vi "test-path-planner-sample.vi"() -> ()   [LabVIEW 2019]
uses:
  <vilib>/Rock Robotics/WPI/ThirdParty/MJansen/PathPlanner/PathPlanner24.lvlib
  <vilib>/Rock Robotics/WPI/ThirdParty/JAS_Junk/TrajLib/Trajectory_Library.lvlib
  <vilib>/Analysis/NI_AALBase.lvlib
  <vilib>/Rock Robotics/WPI/ThirdParty/JAS_Junk/TrajLib/TypeDef/ROTATION2D.ctl
  <vilib>/Rock Robotics/WPI/ThirdParty/JAS_Junk/TrajLib/TypeDef/TRANSLATION2D.ctl
  <vilib>/Rock Robotics/WPI/ThirdParty/MJansen/PathPlanner/TypeDef/PathPlannerTrajectoryState.ctl
  <vilib>/Rock Robotics/WPI/ThirdParty/MJansen/PathPlanner/TypeDef/PathPlannerTrajectory.ctl
  <vilib>/Rock Robotics/WPI/ThirdParty/MJansen/PathPlanner/TypeDef/PathPlannerPathConstraints.ctl
  <vilib>/Rock Robotics/WPI/ThirdParty/JAS_Junk/TrajLib/TypeDef/POSE2D.ctl
  <vilib>/Rock Robotics/WPI/ThirdParty/JAS_Junk/TrajLib/TypeDef/TRAJ_STATE.ctl
  <vilib>/Rock Robotics/WPI/ThirdParty/MJansen/PathPlanner/TypeDef/PathPlannerWaypoint.ctl
panel:
  in  "Tab Control":T1(tab)
  in  "Max Velocity":dbl=3.0
  in  "Max Acceleration":dbl=2.0
  in  "stop":bool
  in  "Reversed":bool
  out "PathPlannerWayPoints":T2[](array[typedef]) {"nextControl"."Y" format="%14.3f"; "nextControl"."X" format="%14.3f"; "anchor"."Y" format="%14.3f"; "anchor"."X" format="%14.3f"; "prevControl"."Y" format="%14.3f"; "prevControl"."X" format="%14.3f"}
  in  "Path FileName":string="C:\\Shares\\github\\PathPlannerLabVIEW\\PathPlannerSandbox\\PathPlannerTestPath\\JIM1.path"
  out "LabVIEW path json read error":errorcluster
  out "PathPlannerTrajectory":T4 {"States"."TargetHolonomicRotation"."SIN" format="%13.4f"; "States"."TargetHolonomicRotation"."COS" format="%13.4f"; "States"."TargetHolonomicRotation"."VALUE" format="%13.4f"; "States"."Heading"."SIN" format="%13.4f"; "States"."Heading"."COS" format="%13.4f"; "States"."Heading"."VALUE" format="%13.4f"; "States"."PositionMeters"."Y" format="%14.3f"; "States"."PositionMeters"."X" format="%14.3f"}
  out "outPathPlannerStates":T5[](array[typedef]) {"TargetHolonomicRotation"."SIN" format="%13.4f"; "TargetHolonomicRotation"."COS" format="%13.4f"; "TargetHolonomicRotation"."VALUE" format="%13.4f"; "Heading"."SIN" format="%13.4f"; "Heading"."COS" format="%13.4f"; "Heading"."VALUE" format="%13.4f"; "PositionMeters"."Y" format="%14.3f"; "PositionMeters"."X" format="%14.3f"}
  in  "index":i32
  out "LabVIEW_TotalTime_Sec":dbl
  out "LabVIEWStateCount":i32
  out "States Check":bool[](array[boolean])
  out "Differences":T8[](array[typedef]) {"POSE"."ROTATION"."SIN" format="%13.4f"; "POSE"."ROTATION"."COS" format="%13.4f"; "POSE"."ROTATION"."VALUE" format="%13.4f"; "POSE"."TRANSLATION"."Y" format="%14.3f"; "POSE"."TRANSLATION"."X" format="%14.3f"}
  out "max time diff":dbl
  out "max vel diff":dbl
  out "max accel diff":dbl
  out "max x diff":dbl
  out "max y diff":dbl
  out "max rot diff rad":dbl
  out "max curvature diff":dbl
  out "vel mean":dbl format="%0.6f"
  out "vel std dev":dbl format="%0.6f"
  out "accel mean":dbl format="%0.6f"
  out "accel std dev":dbl format="%0.6f"
  out "Java and LabVIEW \nwithin tolerance":bool
  out "max accel diff\nindex":i32
  out "max time diff\nindex":i32
  out "Path Samp":T8[](array[typedef]) {"POSE"."ROTATION"."SIN" format="%13.4f"; "POSE"."ROTATION"."COS" format="%13.4f"; "POSE"."ROTATION"."VALUE" format="%13.4f"; "POSE"."TRANSLATION"."Y" format="%14.3f"; "POSE"."TRANSLATION"."X" format="%14.3f"}
  out "LV Samp":T8[](array[typedef]) {"POSE"."ROTATION"."SIN" format="%13.4f"; "POSE"."ROTATION"."COS" format="%13.4f"; "POSE"."ROTATION"."VALUE" format="%13.4f"; "POSE"."TRANSLATION"."Y" format="%14.3f"; "POSE"."TRANSLATION"."X" format="%14.3f"}
  in  "Tolerance":T8={"TimeSeconds"=0.005, "Velocity"=0.005, "Acceleration"=0.2, "POSE"={"TRANSLATION"={"X"=0.002, "Y"=0.002}, "ROTATION"={"VALUE"=0.002, "COS"=0.002, "SIN"=0.002}}, "Curvature"=0.3} {"POSE"."ROTATION"."SIN" format="%13.4f"; "POSE"."ROTATION"."COS" format="%13.4f"; "POSE"."ROTATION"."VALUE" format="%13.4f"; "POSE"."TRANSLATION"."Y" format="%14.3f"; "POSE"."TRANSLATION"."X" format="%14.3f"}
  out "XY SPLINE":cluster{dbl[], dbl[]}[](graph)
  out "XY Graph":cluster{dbl[], dbl[]}[](graph)
  out "Sample Graph":dbl[][](graph)
  out "LabVIEW Time Plot":cluster{dbl[], dbl[]}[](graph)
  out "Diff Time Plot":cluster{dbl[], dbl[]}[](graph)
  in  "PPS2":T5={"TimeSeconds"=4.0, "VelocityMPS"=4.0, "AccerationMpsSq"=4.0, "HeadingAngularVelRadPerSec"=4.0, "PositionMeters"={"X"=1.5, "Y"=0.071}, "Heading"={"VALUE"=1.5, "COS"=0.071, "SIN"=0.997}, "TargetHolonomicRotation"={"VALUE"=0.0, "COS"=1.0, "SIN"=0.0}, "CurvatureRadPerMeter"=4.0, "PathPlannerConstraints"={"MaxVelocityMps;"=2.0, "MaxAccelerationMpsSq;"=4.0, "MaxAngularVelRadPsEc;"=4.0, "MaxAngularAccRadPSecSq"=0.25, "Exists"=FALSE, "Unlimited"=FALSE, "NominalVoltageVolts"=1.5}, "DeltaPos"=2.0} {"TargetHolonomicRotation"."SIN" format="%13.4f"; "TargetHolonomicRotation"."COS" format="%13.4f"; "TargetHolonomicRotation"."VALUE" format="%13.4f"; "Heading"."SIN" format="%13.4f"; "Heading"."COS" format="%13.4f"; "Heading"."VALUE" format="%13.4f"; "PositionMeters"."Y" format="%14.3f"; "PositionMeters"."X" format="%14.3f"}
  in  "PPS1":T5={"TimeSeconds"=2.0, "VelocityMPS"=2.0, "AccerationMpsSq"=2.0, "HeadingAngularVelRadPerSec"=2.0, "PositionMeters"={"X"=0.5, "Y"=0.878}, "Heading"={"VALUE"=0.5, "COS"=0.878, "SIN"=0.479}, "TargetHolonomicRotation"={"VALUE"=0.0, "COS"=1.0, "SIN"=0.0}, "CurvatureRadPerMeter"=2.0, "PathPlannerConstraints"={"MaxVelocityMps;"=1.0, "MaxAccelerationMpsSq;"=2.0, "MaxAngularVelRadPsEc;"=2.0, "MaxAngularAccRadPSecSq"=0.5, "Exists"=FALSE, "Unlimited"=FALSE, "NominalVoltageVolts"=0.5}, "DeltaPos"=1.0} {"TargetHolonomicRotation"."SIN" format="%13.4f"; "TargetHolonomicRotation"."COS" format="%13.4f"; "TargetHolonomicRotation"."VALUE" format="%13.4f"; "Heading"."SIN" format="%13.4f"; "Heading"."COS" format="%13.4f"; "Heading"."VALUE" format="%13.4f"; "PositionMeters"."Y" format="%14.3f"; "PositionMeters"."X" format="%14.3f"}
  in  "PPS0":T5={"TimeSeconds"=1.0, "VelocityMPS"=1.0, "AccerationMpsSq"=1.0, "HeadingAngularVelRadPerSec"=1.0, "PositionMeters"={"X"=0.0, "Y"=1.0}, "Heading"={"VALUE"=0.0, "COS"=1.0, "SIN"=0.0}, "TargetHolonomicRotation"={"VALUE"=0.0, "COS"=1.0, "SIN"=0.0}, "CurvatureRadPerMeter"=1.0, "PathPlannerConstraints"={"MaxVelocityMps;"=0.0, "MaxAccelerationMpsSq;"=1.0, "MaxAngularVelRadPsEc;"=1.0, "MaxAngularAccRadPSecSq"=1.0, "Exists"=FALSE, "Unlimited"=FALSE, "NominalVoltageVolts"=0.0}, "DeltaPos"=1.0} {"TargetHolonomicRotation"."SIN" format="%13.4f"; "TargetHolonomicRotation"."COS" format="%13.4f"; "TargetHolonomicRotation"."VALUE" format="%13.4f"; "Heading"."SIN" format="%13.4f"; "Heading"."COS" format="%13.4f"; "Heading"."VALUE" format="%13.4f"; "PositionMeters"."Y" format="%14.3f"; "PositionMeters"."X" format="%14.3f"}
  out "TrajState":T8={"TimeSeconds"=0.0, "Velocity"=0.0, "Acceleration"=0.0, "POSE"={"TRANSLATION"={"X"=0.0, "Y"=0.0}, "ROTATION"={"VALUE"=0.0, "COS"=1.0, "SIN"=0.0}}, "Curvature"=0.0} {"POSE"."ROTATION"."SIN" format="%13.4f"; "POSE"."ROTATION"."COS" format="%13.4f"; "POSE"."ROTATION"."VALUE" format="%13.4f"; "POSE"."TRANSLATION"."Y" format="%14.3f"; "POSE"."TRANSLATION"."X" format="%14.3f"}
  out "PathState":T8={"TimeSeconds"=0.0, "Velocity"=0.0, "Acceleration"=0.0, "POSE"={"TRANSLATION"={"X"=0.0, "Y"=0.0}, "ROTATION"={"VALUE"=0.0, "COS"=1.0, "SIN"=0.0}}, "Curvature"=0.0} {"POSE"."ROTATION"."SIN" format="%13.4f"; "POSE"."ROTATION"."COS" format="%13.4f"; "POSE"."ROTATION"."VALUE" format="%13.4f"; "POSE"."TRANSLATION"."Y" format="%14.3f"; "POSE"."TRANSLATION"."X" format="%14.3f"}
  out "LabVIEWStates":T8[](array[typedef]) {"POSE"."ROTATION"."SIN" format="%13.4f"; "POSE"."ROTATION"."COS" format="%13.4f"; "POSE"."ROTATION"."VALUE" format="%13.4f"; "POSE"."TRANSLATION"."Y" format="%14.3f"; "POSE"."TRANSLATION"."X" format="%14.3f"}
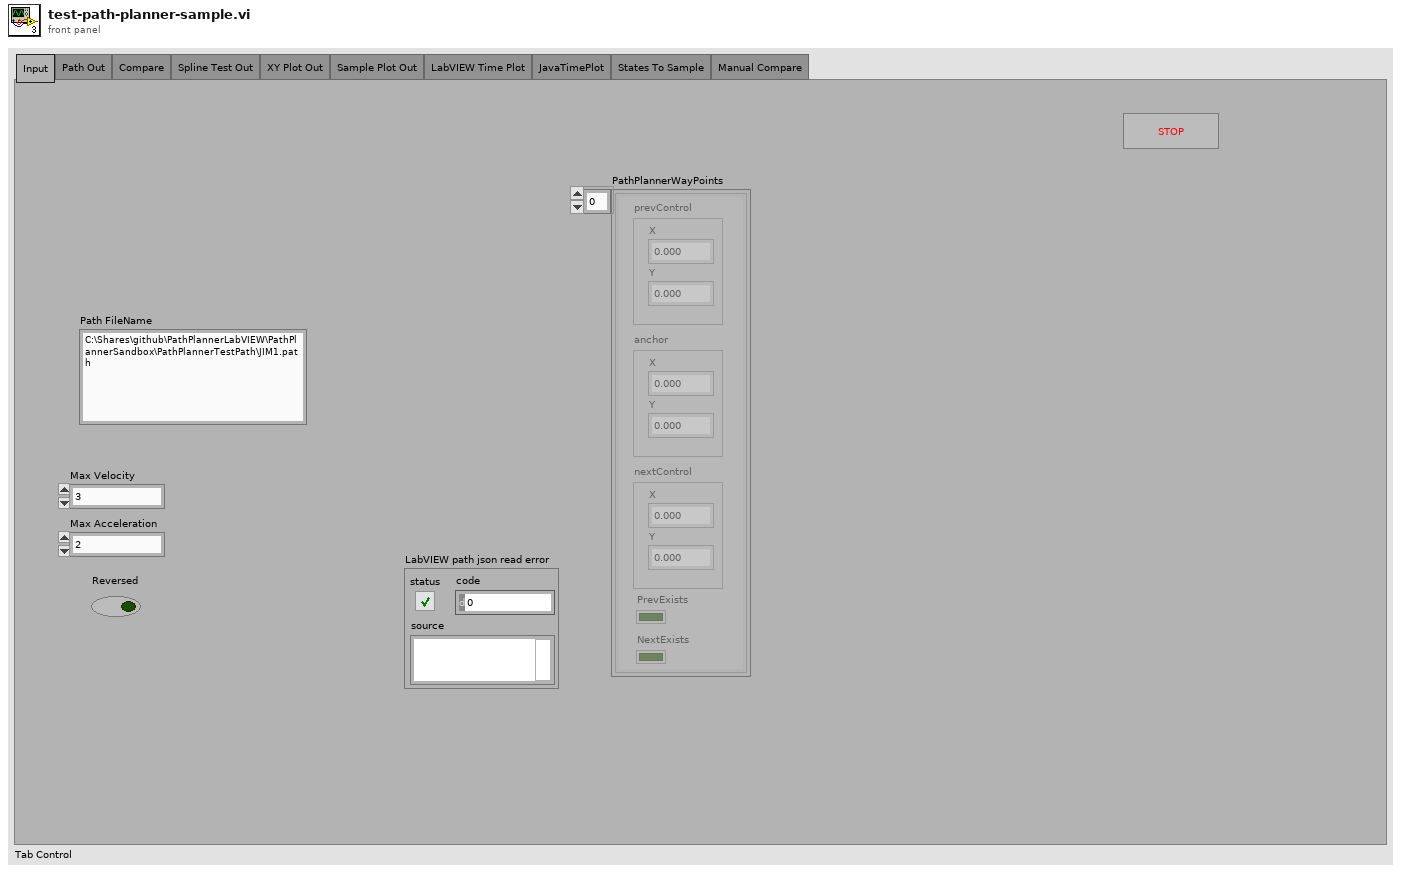
[diagram p1: front panel]
types:
  T1 = enum32{"Input", "Path Out", "Compare", "Spline Test Out", "XY Plot Out", "Sample Plot Out", "LabVIEW Time Plot", "JavaTimePlot", "States To Sample", "Manual Compare"}
  T2 = typedef "PathPlanner24.lvlib/PathPlannerWaypoint.ctl" = cluster{"prevControl":T3, "anchor":T3, "nextControl":T3, "PrevExists":bool, "NextExists":bool}
  T3 = typedef "Trajectory_Library.lvlib/TRANSLATION2D.ctl" = cluster{"X":dbl, "Y":dbl}
  T4 = typedef "PathPlanner24.lvlib/PathPlannerTrajectory.ctl" = cluster{"States":T5[]}
  T5 = typedef "PathPlanner24.lvlib/PathPlannerTrajectoryState.ctl" = cluster{"TimeSeconds":dbl, "VelocityMPS":dbl, "AccerationMpsSq":dbl, "HeadingAngularVelRadPerSec":dbl, "PositionMeters":T3, "Heading":T6, "TargetHolonomicRotation":T6, "CurvatureRadPerMeter":dbl, "PathPlannerConstraints":T7, "DeltaPos":dbl}
  T6 = typedef "Trajectory_Library.lvlib/ROTATION2D.ctl" = cluster{"VALUE":dbl, "COS":dbl, "SIN":dbl}
  T7 = typedef "PathPlanner24.lvlib/PathPlannerPathConstraints.ctl" = cluster{"MaxVelocityMps;":dbl, "MaxAccelerationMpsSq;":dbl, "MaxAngularVelRadPsEc;":dbl, "MaxAngularAccRadPSecSq":dbl, "Exists":bool, "Unlimited":bool, "NominalVoltageVolts":dbl}
  T8 = typedef "Trajectory_Library.lvlib/TRAJ_STATE.ctl" = cluster{"TimeSeconds":dbl, "Velocity":dbl, "Acceleration":dbl, "POSE":T9, "Curvature":dbl}
  T9 = typedef "Trajectory_Library.lvlib/POSE2D.ctl" = cluster{"TRANSLATION":T3, "ROTATION":T6}
  T10 = typedef "Trajectory_Library.lvlib/TRAJECTORY.ctl" = cluster{"TotalTImeSecs":dbl, "States":T8[]}
  T11 = typedef "PathPlanner24.lvlib/PathPlannerPath.ctl" = cluster{"Reversed":bool, "RotationTargets":T12[], "ConstraintZones":T13[], "EventMarkers":T14[], "GlobalConstraints":T7, "GoalEndState":T17, "AllPoints":T18[], "Name":string, "Waypoints":T2[], "PointTowardsZones":T19[], "IdealStartingState":T20, "IsChoreoPath":bool, "PreventFlipping":bool}
  T12 = typedef "PathPlanner24.lvlib/PathPlannerRotationTarget.ctl" = cluster{"position":dbl, "rotation":T6, "Exists":bool}
  T13 = typedef "PathPlanner24.lvlib/PathPlannerConstraintsZone.ctl" = cluster{"minPosition":dbl, "maxPosition":dbl, "Constraints":T7, "Present":bool}
  T14 = typedef "PathPlanner24.lvlib/PathPlannerEventMarker.ctl" = cluster{"Position":dbl, "Command":T15, "TriggerName":string, "EndPosition":dbl}
  T15 = typedef "PathPlanner24.lvlib/PathPlannerCommandUtil.ctl" = cluster{"waitTime":dbl, "name":string, "pathName":string, "commands":cluster{"type":T16, "waitTime":dbl, "name":string, "pathName":string}[], "type":T16}
  T16 = typedef "PathPlanner24.lvlib/PathPlanner_CommandUtilType_ENUM.ctl" = enum16{"Unknown", "Wait", "Named", "Path", "Sequential", "Parallel", "Race", "Deadline"}
  T17 = typedef "PathPlanner24.lvlib/PathPlannerGoalEndState.ctl" = cluster{"VelocityMPS":dbl, "Rotation":T6}
  T18 = typedef "PathPlanner24.lvlib/PathPlannerPathPoint.ctl" = cluster{"Position":T3, "DistAlongPath":dbl, "MaxV":dbl, "Constraints":T7, "RotationTarget":T12, "WaypointRelativePos":dbl}
  T19 = typedef "PathPlanner24.lvlib/PathPlannerPointTowardsZone.ctl" = cluster{"RotationOffset":T6, "Name":string, "TargetPosition":T3, "MinPosition":dbl, "MaxPosition":dbl}
  T20 = typedef "PathPlanner24.lvlib/PathPlannerIdealStartingState.ctl" = cluster{"VelocityMPS":dbl, "Rotation":T6}
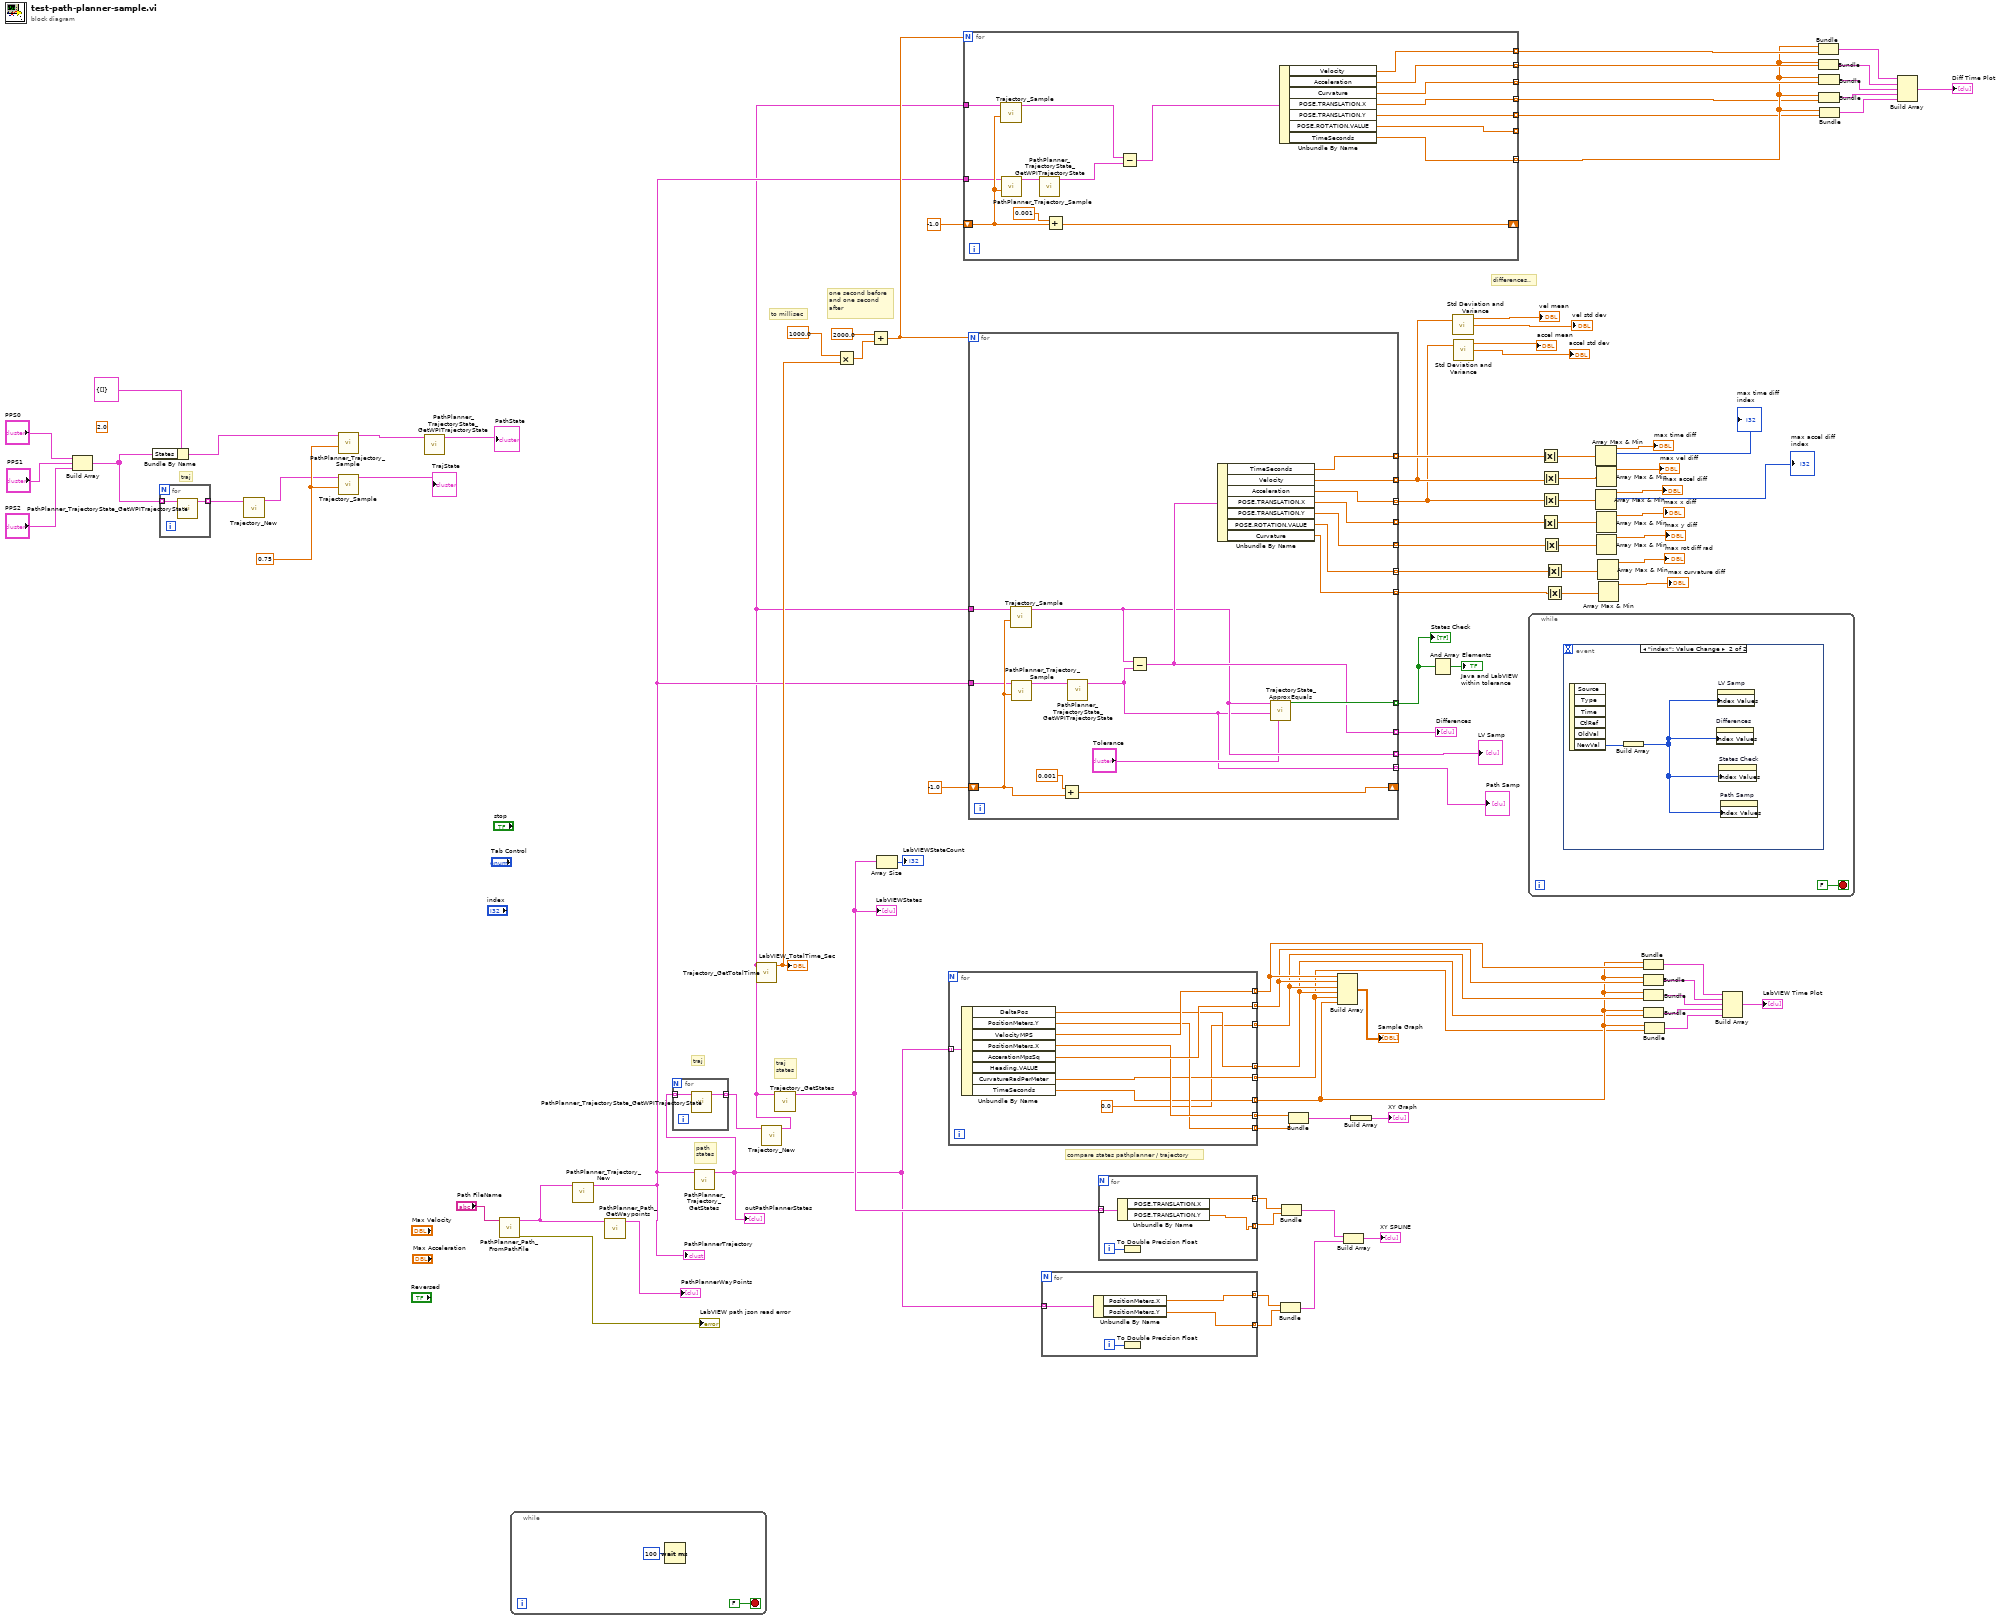
[diagram p0: block diagram]
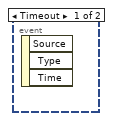
[diagram p2: hidden frame]
diagram:
  w18 = 0.75
  (unwired) 2.0 ("TotalTimeSeconds")
  # "traj"
  # "one second before\nand one second\nafter"
  # "to millisec"
  # "compare states pathplanner / trajectory"
  # "traj"
  # "traj\nstates"
  # "path\nstates"
  # "differences.."
  n1 = Build Array("PPS0", "PPS1", "PPS2") -> (w5:T5[])
  n2 = Bundle By Name(cluster=T4 {"States"=[]} ("PathPlannerTrajectory"), "States"=w5) -> (w6:T4)
  n3 = for {
    tunnel: w5 -> [w99] mode=indexing
    tunnel: [w98] -> w4 mode=indexing
    n4 = call <vilib>:"PathPlanner_TrajectoryState_GetWPITrajectoryState.vi"("PathPlannerState"=w99) -> ("WPI TrajectoryState"=w98:T8)  [unwired: 9 in, 1 out]
  }
  n5 = call <vilib>:"Trajectory_New.vi"("TRAJ_STATES"=w4) -> ("TRAJECTORY"=w3:T10)  [unwired: 10 in]
  n6 = call <vilib>:"PathPlanner_Trajectory_Sample.vi"("Time"=w18, "PathPlannerTrajectory"=w6) -> ("PathPlannerState"=w2:T5)  [unwired: 9 in]
  n7 = call <vilib>:"Trajectory_Sample.vi"("Time"=w18, "InputTRAJECTORY"=w3) -> ("OutputTRAJ_STATE"=→"TrajState":T8)  [unwired: 9 in]
  n8 = call <vilib>:"PathPlanner_TrajectoryState_GetWPITrajectoryState.vi"("PathPlannerState"=w2) -> ("WPI TrajectoryState"=→"PathState":T8)  [unwired: 9 in, 1 out]
  n9 = call <vilib>:"PathPlanner_Path_FromPathFile.vi"("FileName"="Path FileName") -> ("error out"=→"LabVIEW path json read error":errorcluster, "PathPlannerPath"=w11:T11)  [unwired: 7 in, 2 out]
  n10 = while {
    stop <- FALSE stop-if-true
    n11 = Wait (ms)(milliseconds to wait=u32 100) -> ()  [unwired: 1 out]
  }
  n12 = call <vilib>:"PathPlanner_Trajectory_New.vi"("Path"=w11) -> ("PathPlannerTrajectory"=w12:T4)  [unwired: 9 in, 1 out]
  "PathPlannerTrajectory" <- w12
  n13 = call <vilib>:"PathPlanner_Path_GetWaypoints.vi"("PathPlannerPath"=w11) -> ("Waypoints"=→"PathPlannerWayPoints":T2[])  [unwired: 10 in]
  n14 = call <vilib>:"PathPlanner_Trajectory_GetStates.vi"("PathPlannerTrajectory"=w12) -> ("PathPlannerStates"=w9:T5[])  [unwired: 10 in]
  "outPathPlannerStates" <- w9
  n15 = for {
    tunnel: w9 -> [w103] mode=indexing
    tunnel: [w102] -> w8 mode=indexing
    n16 = call <vilib>:"PathPlanner_TrajectoryState_GetWPITrajectoryState.vi"("PathPlannerState"=w103) -> ("WPI TrajectoryState"=w102:T8)  [unwired: 9 in, 1 out]
  }
  n17 = call <vilib>:"Trajectory_New.vi"("TRAJ_STATES"=w8) -> ("TRAJECTORY"=w7:T10)  [unwired: 10 in]
  n18 = call <vilib>:"Trajectory_GetTotalTime.vi"("TRAJECTORY"=w7) -> ("TotalTime_Sec"=w40:dbl)  [unwired: 10 in]
  "LabVIEW_TotalTime_Sec" <- w40
  n19 = call <vilib>:"Trajectory_GetStates.vi"("TRAJECTORY"=w7) -> ("States"=w41:T8[])  [unwired: 10 in]
  "LabVIEWStates" <- w41
  n20 = Multiply(x=1000.0, y=w40) -> (x*y=w44:dbl)
  n21 = Add(x=2000.0, y=w44) -> (x+y=w39:dbl)
  n22 = Array Size(array=w41) -> (size(s)=→"LabVIEWStateCount":i32)
  n23 = for {
    tunnel: [w112] -> w70 mode=indexing
    tunnel: [w111] -> w69 mode=indexing
    tunnel: [w106] -> w66 mode=indexing
    tunnel: [w110] -> w96 mode=indexing
    tunnel: [w109] -> w95 mode=indexing
    tunnel: w9 -> [w108] mode=indexing
    tunnel: [w107] -> w65 mode=indexing
    tunnel: [0.0] -> w68 mode=indexing
    tunnel: [w105] -> w67 mode=indexing
    n24 = Unbundle By Name(w108) -> ("DeltaPos"=w106:dbl, "PositionMeters.Y"=w109:dbl, "VelocityMPS"=w112:dbl, "PositionMeters.X"=w110:dbl, "AccerationMpsSq"=w111:dbl, "CurvatureRadPerMeter"=w107:dbl, "TimeSeconds"=w105:dbl)  [unwired: 1 out]
  }
  n25 = for {
    N: w39 -> [_]
    tunnel: [w120] -> w59 mode=indexing
    tunnel: [w119] -> w58 mode=indexing
    tunnel: [w117] -> w55 mode=indexing
    tunnel: [w116] -> w54 mode=indexing
    tunnel: [w118] -> w57 mode=indexing
    tunnel: [w128] -> w56 mode=indexing
    shift-right: [w124] -> _
    shift-left: -1.0 -> [w123]
    tunnel: w12 -> [w122]
    tunnel: w7 -> [w121]
    tunnel: [w115] -> _ mode=indexing
    n26 = call <vilib>:"Trajectory_Sample.vi"("Time"=w123, "InputTRAJECTORY"=w121) -> ("OutputTRAJ_STATE"=w127:T8)  [unwired: 9 in]
    n27 = call <vilib>:"PathPlanner_Trajectory_Sample.vi"("Time"=w123, "PathPlannerTrajectory"=w122) -> ("PathPlannerState"=w114:T5)  [unwired: 9 in]
    n28 = call <vilib>:"PathPlanner_TrajectoryState_GetWPITrajectoryState.vi"("PathPlannerState"=w114) -> ("WPI TrajectoryState"=w113:T8)  [unwired: 9 in, 1 out]
    n29 = Add(x=0.001, y=w123) -> (x+y=w124:dbl)
    n30 = Subtract(x=w127, y=w113) -> (x-y=w126:T8)
    n31 = Unbundle By Name(w126) -> ("Velocity"=w120:dbl, "Acceleration"=w119:dbl, "Curvature"=w118:dbl, "POSE.TRANSLATION.X"=w117:dbl, "POSE.TRANSLATION.Y"=w116:dbl, "POSE.ROTATION.VALUE"=w115:dbl, "TimeSeconds"=w128:dbl)
  }
  n32 = for {
    N: w39 -> [_]
    tunnel: [w146] -> w48 mode=indexing
    tunnel: [w145] -> w37 mode=indexing
    tunnel: [w144] -> w24 mode=indexing
    tunnel: [w143] -> w23 mode=indexing
    tunnel: [w142] -> w36 mode=indexing
    tunnel: [w141] -> w35 mode=indexing
    tunnel: [w140] -> w34 mode=indexing
    tunnel: [w139] -> w33 mode=indexing
    shift-right: [w137] -> _
    shift-left: -1.0 -> [w136]
    tunnel: w12 -> [w135]
    tunnel: w7 -> [w134]
    tunnel: [w133] -> w25 mode=indexing
    tunnel: [w132] -> w14 mode=indexing
    tunnel: [w129] -> w13 mode=indexing
    n33 = call <vilib>:"Trajectory_Sample.vi"("Time"=w136, "InputTRAJECTORY"=w134) -> ("OutputTRAJ_STATE"=w132:T8)  [unwired: 9 in]
    n34 = call <vilib>:"PathPlanner_Trajectory_Sample.vi"("Time"=w136, "PathPlannerTrajectory"=w135) -> ("PathPlannerState"=w130:T5)  [unwired: 9 in]
    n35 = Add(x=0.001, y=w136) -> (x+y=w137:dbl)
    n36 = call <vilib>:"PathPlanner_TrajectoryState_GetWPITrajectoryState.vi"("PathPlannerState"=w130) -> ("WPI TrajectoryState"=w129:T8)  [unwired: 9 in, 1 out]
    n37 = Subtract(x=w132, y=w129) -> (x-y=w133:T8)
    n38 = Unbundle By Name(w133) -> ("TimeSeconds"=w145:dbl, "Velocity"=w144:dbl, "Acceleration"=w143:dbl, "POSE.TRANSLATION.X"=w142:dbl, "POSE.TRANSLATION.Y"=w141:dbl, "POSE.ROTATION.VALUE"=w140:dbl, "Curvature"=w139:dbl)
    n39 = call "TrajectoryState_ApproxEquals.vi"("Tolerance"="Tolerance", "Other TRAJ_STATE"=w129, "TRAJ_STATE"=w132) -> ("Equals"=w146:bool)  [unwired: 8 in]
  }
  "States Check" <- w48
  "Differences" <- w25
  "LV Samp" <- w14
  "Path Samp" <- w13
  n40 = for {
    tunnel: [w149] -> w90 mode=indexing
    tunnel: w9 -> [w148] mode=indexing
    tunnel: [w147] -> w89 mode=indexing
    i -> [w150]
    n41 = Unbundle By Name(w148) -> ("PositionMeters.X"=w149:dbl, "PositionMeters.Y"=w147:dbl)
    n42 = To Double Precision Float(number=w150) -> ()  [unwired: 1 out]
  }
  n43 = for {
    tunnel: [w153] -> w92 mode=indexing
    tunnel: [w152] -> w91 mode=indexing
    tunnel: w41 -> [w151] mode=indexing
    i -> [w154]
    n44 = Unbundle By Name(w151) -> ("POSE.TRANSLATION.X"=w153:dbl, "POSE.TRANSLATION.Y"=w152:dbl)
    n45 = To Double Precision Float(number=w154) -> ()  [unwired: 1 out]
  }
  n46 = Bundle(w90, w89) -> (w87:cluster{dbl[], dbl[]})  [unwired: 1 in]
  n47 = Bundle(w92, w91) -> (w88:cluster{dbl[], dbl[]})  [unwired: 1 in]
  n48 = Bundle(w96, w95) -> (w94:cluster{dbl[], dbl[]})  [unwired: 1 in]
  n49 = Build Array(w70, w69, w68, w66, w65, w67) -> (→"Sample Graph":dbl[][])
  n50 = Build Array(w88, w87) -> (→"XY SPLINE":cluster{dbl[], dbl[]}[])
  n51 = Build Array(w94) -> (→"XY Graph":cluster{dbl[], dbl[]}[])
  n52 = And Array Elements(Boolean array=w48) -> (logical AND=→"Java and LabVIEW \nwithin tolerance":bool)
  n53 = call <vilib>:"Std Deviation and Variance.vi"("X"=w24) -> ("mean"=→"vel mean":dbl, "standard deviation"=→"vel std dev":dbl)  [unwired: 1 in, 1 out]
  n54 = call <vilib>:"Std Deviation and Variance.vi"("X"=w23) -> ("mean"=→"accel mean":dbl, "standard deviation"=→"accel std dev":dbl)  [unwired: 1 in, 1 out]
  n55 = while {
    stop <- FALSE stop-if-true
    n56 = event shown="[1] \"index\": Value Change" {
      selector: _ -> [_ _]
      dyn-events: _ -> [_ _]
      timeout: _ -> [_ _]
      event Timeout {
        n57 = event-data() -> ()  [unwired: 1 in, 3 out]
      }
      event "index": Value Change {
        n58 = event-data() -> ("NewVal"=w157:i32)  [unwired: 1 in, 5 out]
        n59 = Build Array(w157) -> (w156:i32[])
        n60 = property on="Differences" class="Arr (strict)"("Index Values"=w156) -> ()  [unwired: 2 in, 2 out]
        n61 = property on="LV Samp" class="Arr (strict)"("Index Values"=w156) -> ()  [unwired: 2 in, 2 out]
        n62 = property on="States Check" class="Arr (strict)"("Index Values"=w156) -> ()  [unwired: 2 in, 2 out]
        n63 = property on="Path Samp" class="Arr (strict)"("Index Values"=w156) -> ()  [unwired: 2 in, 2 out]
      }
    }
  }
  n64 = Absolute Value(x=w37) -> (abs(x)=w32:dbl[])
  n65 = Absolute Value(x=w36) -> (abs(x)=w29:dbl[])
  n66 = Absolute Value(x=w24) -> (abs(x)=w31:dbl[])
  n67 = Absolute Value(x=w23) -> (abs(x)=w30:dbl[])
  n68 = Absolute Value(x=w35) -> (abs(x)=w28:dbl[])
  n69 = Absolute Value(x=w34) -> (abs(x)=w27:dbl[])
  n70 = Absolute Value(x=w33) -> (abs(x)=w26:dbl[])
  n71 = Array Max & Min(array=w32) -> (max value=→"max time diff":dbl, max index (indices)=→"max time diff\nindex":i32)  [unwired: 2 out]
  n72 = Array Max & Min(array=w30) -> (max value=→"max accel diff":dbl, max index (indices)=→"max accel diff\nindex":i32)  [unwired: 2 out]
  n73 = Array Max & Min(array=w31) -> (max value=→"max vel diff":dbl)  [unwired: 3 out]
  n74 = Array Max & Min(array=w29) -> (max value=→"max x diff":dbl)  [unwired: 3 out]
  n75 = Array Max & Min(array=w28) -> (max value=→"max y diff":dbl)  [unwired: 3 out]
  n76 = Array Max & Min(array=w27) -> (max value=→"max rot diff rad":dbl)  [unwired: 3 out]
  n77 = Array Max & Min(array=w26) -> (max value=→"max curvature diff":dbl)  [unwired: 3 out]
  n78 = Bundle(w67, w70) -> (w64:cluster{dbl[], dbl[]})  [unwired: 1 in]
  n79 = Bundle(w67, w69) -> (w63:cluster{dbl[], dbl[]})  [unwired: 1 in]
  n80 = Bundle(w67, w68) -> (w62:cluster{dbl[], dbl[]})  [unwired: 1 in]
  n81 = Bundle(w67, w66) -> (w61:cluster{dbl[], dbl[]})  [unwired: 1 in]
  n82 = Bundle(w67, w65) -> (w60:cluster{dbl[], dbl[]})  [unwired: 1 in]
  n83 = Build Array(w64, w63, w62, w61, w60) -> (→"LabVIEW Time Plot":cluster{dbl[], dbl[]}[])
  n84 = Bundle(w56, w59) -> (w53:cluster{dbl[], dbl[]})  [unwired: 1 in]
  n85 = Bundle(w56, w58) -> (w52:cluster{dbl[], dbl[]})  [unwired: 1 in]
  n86 = Bundle(w56, w57) -> (w51:cluster{dbl[], dbl[]})  [unwired: 1 in]
  n87 = Bundle(w56, w55) -> (w50:cluster{dbl[], dbl[]})  [unwired: 1 in]
  n88 = Bundle(w56, w54) -> (w49:cluster{dbl[], dbl[]})  [unwired: 1 in]
  n89 = Build Array(w53, w52, w51, w50, w49) -> (→"Diff Time Plot":cluster{dbl[], dbl[]}[])
